vi "Create NEW Folder.vi"(0 "Base Path":path, 2 "NEW Folder Name":string, 5 "error in (no error)":errorcluster) -> (14 "NEW Folder Path":path, 19 "error out":errorcluster)   [LabVIEW 2022 SP3, in "Generic Utilities.lvclass"]
uses:
  Generic Utilities.lvclass
  <vilib>/Utility/sysdir.llb/System Directory Type.ctl
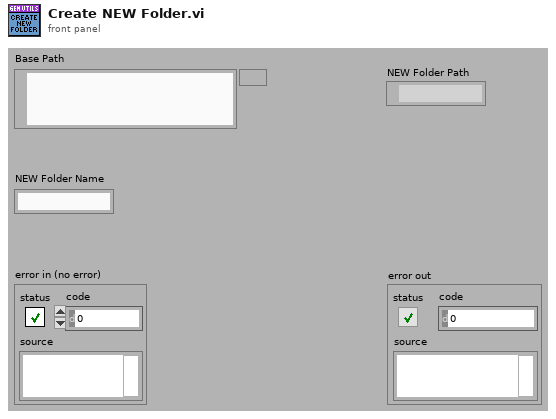
[diagram p1: front panel]
types:
  T1 = typedef "System Directory Type.ctl" = i32
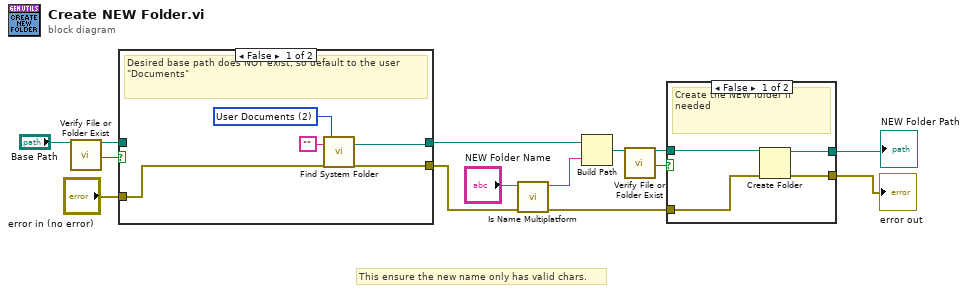
[diagram p0: block diagram]
diagram:
  # "This ensure the new name only has valid chars."
  n1 = call "Verify File or Folder Exist.vi"("path"="Base Path") -> ("dup path"=w11:path, "file or folder exists?"=w12:bool)  [unwired: 16 in, 1 out]
  n2 = case shown="False" w12 {
    tunnel: [w18 w21] -> w8
    tunnel: w11 -> [_ w21]
    tunnel: "error in (no error)" -> [w16 w20]
    tunnel: [w15 w20] -> w9
    frame False {
      w19 = T1 2 items=["User Home"=0, "User Desktop"=1, "User Documents"=2, "User Application Data"=3, "User Preferences"=4, "User Temporary"=5, "Public Documents"=6, "Public Application Data"=7, "Public Preferences"=8, "Public Cache"=13, "System Core Libraries"=9, "System Installed Libraries"=10, "Application Files"=11, "Boot Volume Root"=12] ("system directory type")
      # "Desired base path does NOT exist, so default to the user \"Documents\""
      n3 = call "Find System Folder.vi"("Application Name"="", "error in (no error)"=w16, "system directory type"=w19) -> ("System Folder"=w18:path, "error out"=w15:errorcluster)  [unwired: 15 in]
    }
    frame True {
      # "Desired base path is available, everything is OK"
    }
  }
  n4 = call <vilib>:"Is Name Multiplatform.vi"("error in (no error)"=w9, "filename"="NEW Folder Name") -> ("error out"=w1:errorcluster, "suggested filename"=w7:string)  [unwired: 5 in, 3 out]
  n5 = Build Path(base path=w8, name or relative path=w7) -> (appended path=w4:path)
  n6 = call "Verify File or Folder Exist.vi"("path"=w4) -> ("dup path"=w2:path, "file or folder exists?"=w3:bool)  [unwired: 16 in, 1 out]
  n7 = case shown="False" w3 {
    tunnel: [w25 w27] -> w6
    tunnel: [w24 w26] -> w5
    tunnel: w2 -> [w23 w27]
    tunnel: w1 -> [w22 w26]
    frame False {
      # "Create the NEW folder if needed"
      n8 = Create Folder(path (use dialog)=w23, error in=w22) -> (created path=w25:path, error out=w24:errorcluster)  [unwired: 1 in, 1 out]
    }
    frame True {
      # "Folder Already exist, do nothing"
    }
  }
  "NEW Folder Path" <- w6
  "error out" <- w5
